vi "Remove from Subpanel.vi"(8 "Error In":errorcluster, 11 "Subpanel Inserter":refnum<class "Subpanel Inserter.lvclass">) -> (0 "error out":errorcluster, 3 "Subpanel Inserter 2":refnum<class "Subpanel Inserter.lvclass">)   [LabVIEW 2014, in "Subpanel Insertion.lvlib" / "Subpanel Inserter.lvclass"]
uses:
  Subpanel Inserter.lvclass
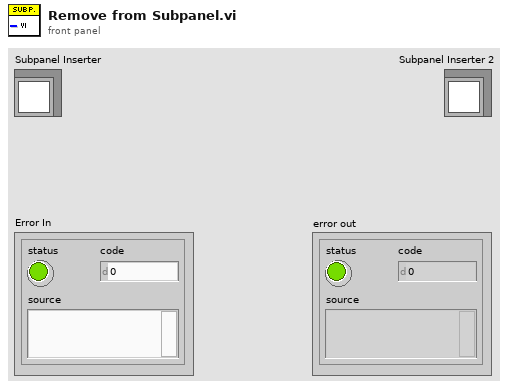
[diagram p1: front panel]
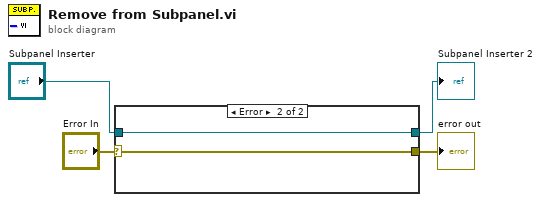
[diagram p0: block diagram]
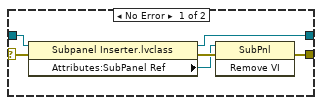
[diagram p2: hidden frame]
diagram:
  n1 = case shown="Error" "Error In" {
    selector: "Error In" -> [w7 w12]
    tunnel: [w10 w12] -> w3
    tunnel: "Subpanel Inserter" -> [w9 w11]
    tunnel: [w5 w11] -> w1
    frame No Error {
      n2 = property class="Subpanel Inserter.lvclass"(reference=w9, error in=w7) -> (reference out=w5:refnum<class "Subpanel Inserter.lvclass">, error out=w8:errorcluster, "Attributes:SubPanel Ref"=w6:refnum<vi>)
      n3 = invoke on="Invoke Node" class="SubPnl" method="Remove VI"(reference=w6, error in=w8) -> (error out=w10:errorcluster)  [unwired: 1 in, 2 out]
    }
    frame Error {
    }
  }
  "error out" <- w3
  "Subpanel Inserter 2" <- w1
